vi "q1.vi"() -> ()   [LabVIEW 2018]
uses:
  Control 5.ctl
  Control 6.ctl
  Control 7.ctl
  <vilib>/measure/NI_MABase.lvlib
panel:
  out "km(t)":dynamicdata(graph)
  out "Waveform Graph":dynamicdata(graph)
  in  "seed":i32=-1
  in  "amplitude":dbl=1.0 format="%0.2p"
  in  "sampling info":cluster{"Fs":T1, "#s":T2}={"Fs"=1000.0, "#s"=1000.0} {"Fs" format="%.2p"}
  in  "frequency":T3=10.0 format="%0.2p"
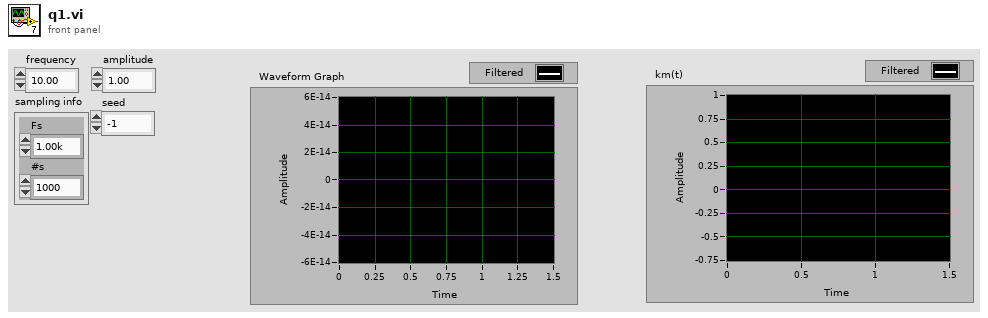
[diagram p1: front panel]
types:
  T1 = typedef "Control 6.ctl" = dbl
  T2 = typedef "Control 7.ctl" = dbl
  T3 = typedef "Control 5.ctl" = dbl
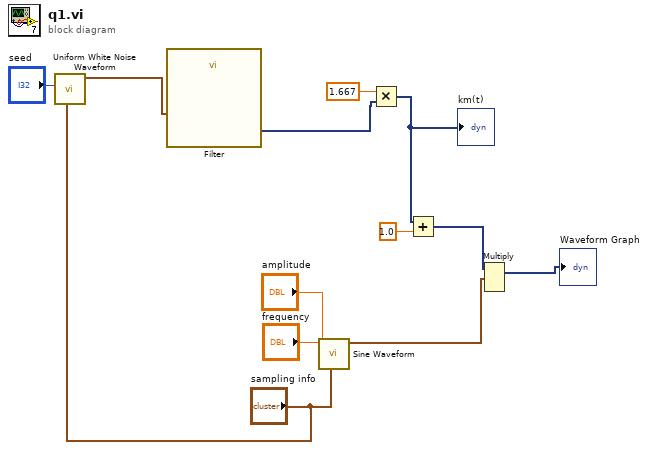
[diagram p0: block diagram]
diagram:
  n1 = call <vilib>:"Uniform White Noise Waveform.vi"("sampling info"="sampling info", "seed"="seed") -> ("signal out"=w12:waveform(dbl))  [unwired: 8 in, 1 out]
  n2 = call "Filter"("Signal"=w12) -> ("Filtered Signal"=w11:dynamicdata)  [unwired: 9 in, 1 out]
  n3 = call <vilib>:"Sine Waveform.vi"("sampling info"="sampling info", "amplitude"="amplitude", "frequency"="frequency") -> ("signal out"=w8:waveform(dbl))  [unwired: 7 in, 1 out]
  n4 = Multiply(x=1.667, y=w11) -> (x*y=w1:dynamicdata)
  "km(t)" <- w1
  n5 = Add(x=w1, y=1.0) -> (x+y=w9:dynamicdata)
  n6 = Multiply(1:w8, 2:w9) -> (0:→"Waveform Graph":dynamicdata)  [unwired: 1 in, 1 out]
